vi "ExposeSetObjectMapNamepathDataToVartiant.vi"(0 "Value In (or type, reference)":refnum<data-value>, 1 "MatlabDataBundle":T1, 2 "NamePath":string[](array[string]), 3 "Namepath Index":i32, 4 "Updatied controls(s)":refnum<vi>[](array[refnum]), 6 "Allow Variant Values (f)":bool, 18 "Info":string[](array[string])) -> (14 "Value Out Ref":refnum<data-value>, 16 "Updated control(s) out":refnum<vi>[](array[refnum]))   [LabVIEW 2017]
uses:
  ExposeObjectMapNamepathData.ctl
  ExposeMapperDataTypeEnum.ctl
  ExposeObjectMapContainerTypeEnum.ctl
panel:
  out "Updating index":i32
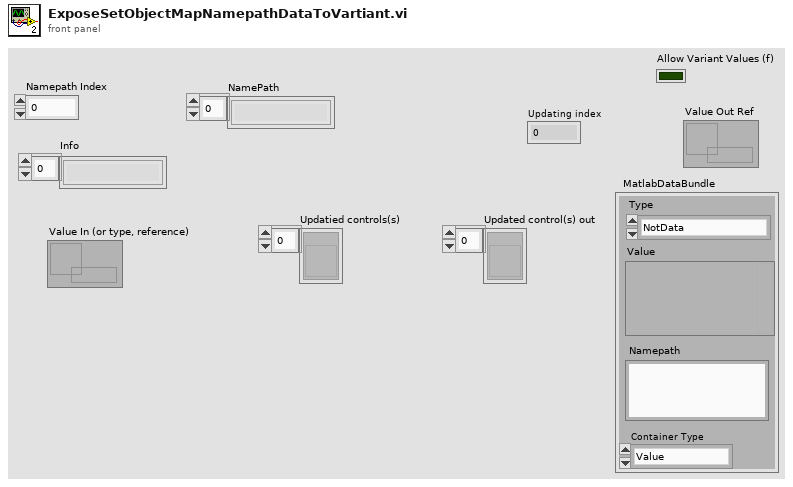
[diagram p1: front panel]
types:
  T1 = typedef "ExposeObjectMapNamepathData.ctl" = cluster{"Type":T2, "Value":variant, "Namepath":string, "Container Type":T3}
  T2 = typedef "ExposeMapperDataTypeEnum.ctl" = enum16{"NotData", "int8", "byte", "int16", "uint16", "int32", "uint32", "int64", "uint64", "Single", "Double", "String", "Boolean", "Container"}
  T3 = typedef "ExposeObjectMapContainerTypeEnum.ctl" = enum16{"Value", "Array", "Waveform", "NetContainer"}
  T4 = typedef "ExposeMapperObjectTypeEnum.ctl" = enum16{"NotAValidObject", "Value", "Variant", "Cluster", "Array", "Asng. Refnum"}
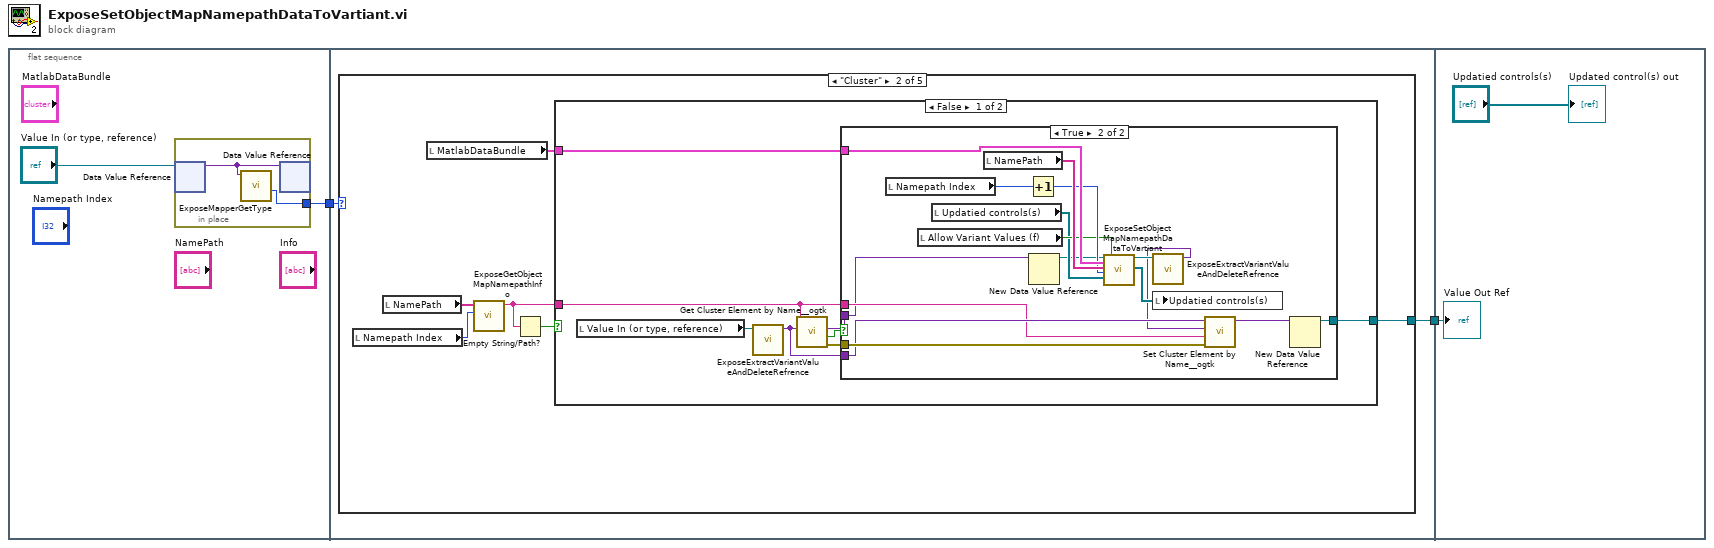
[diagram p0: block diagram]
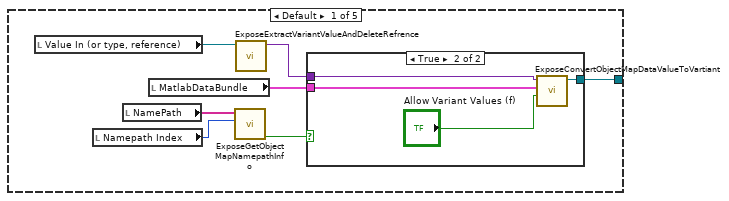
[diagram p2: hidden frame]
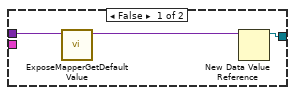
[diagram p3: hidden frame]
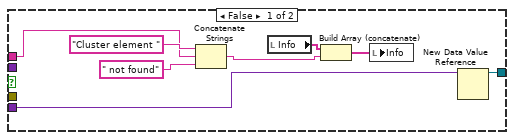
[diagram p4: hidden frame]
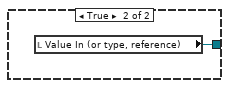
[diagram p5: hidden frame]
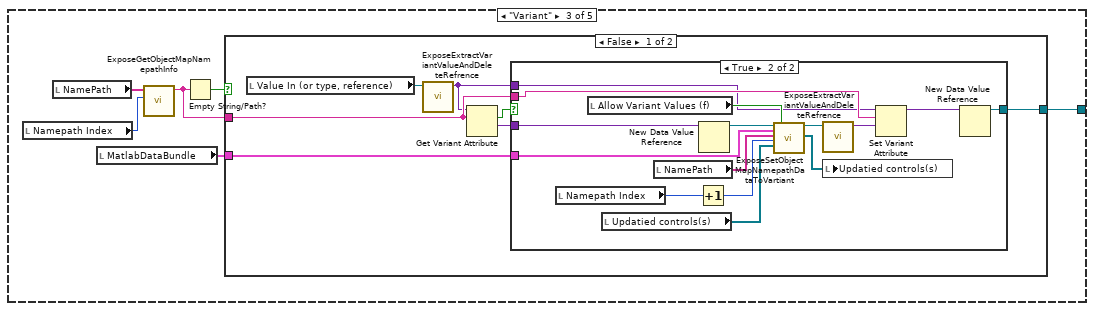
[diagram p6: hidden frame]
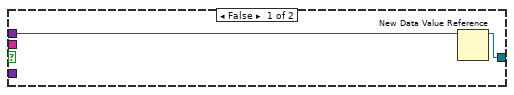
[diagram p7: hidden frame]
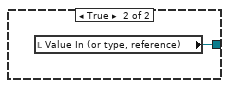
[diagram p8: hidden frame]
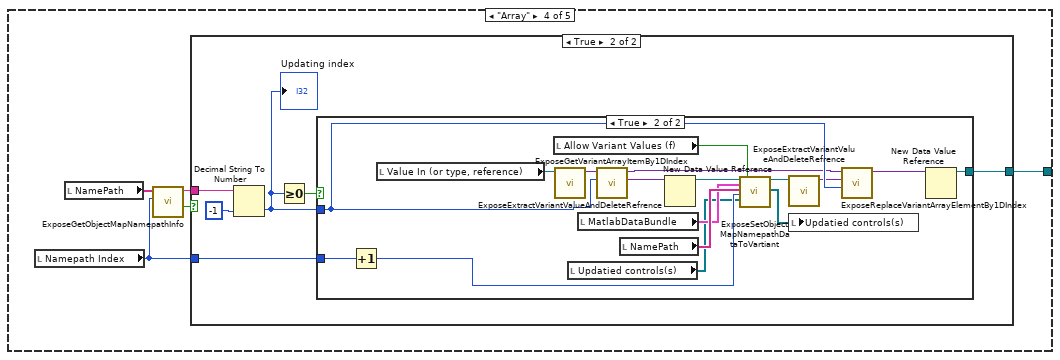
[diagram p9: hidden frame]
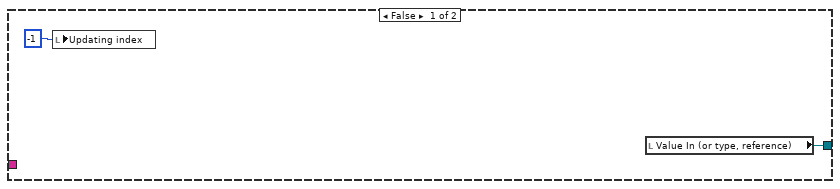
[diagram p10: hidden frame]
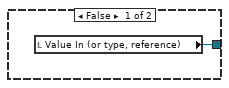
[diagram p11: hidden frame]
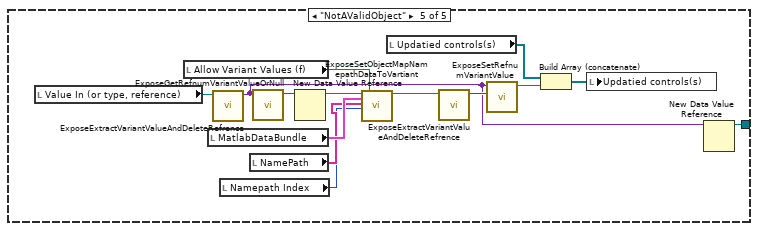
[diagram p12: hidden frame]
diagram:
  n1 = flat-sequence {
    tunnel: [w3] -> w2
    tunnel: w2 -> [w8]
    tunnel: [w7] -> w1
    tunnel: w1 -> [w138]
    frame #0 {
      n2 = in-place {
        in-place-border: [w6] -> w3
        n3 = in-place-dvr #1("Value In (or type, reference)") -> (w5:variant)  [unwired: 1 out]
        n4 = call "ExposeMapperGetType.vi"("Value"=w5) -> ("OType"=w6:T4)  [unwired: 5 in, 5 out]
        n5 = in-place-dvr #1(w5) -> ()  [unwired: 2 out]
      }
    }
    frame #1 {
      n6 = case shown="\"Cluster\"" w8 {
        tunnel: [w11 w23 w62 w93 w126] -> w7
        frame Default {
          n7 = local read "Value In (or type, reference)"() -> (w10:refnum<data-value>)
          n8 = local read "Namepath Index"() -> (w14:i32)
          n9 = local read "NamePath"() -> (w13:string[])
          n10 = local read "MatlabDataBundle"() -> (w15:T1)
          n11 = call "ExposeGetObjectMapNamepathInfo.vi"("Namepath Index"=w14, "NamePath"=w13) -> ("At path end"=w12:bool)  [unwired: 7 in, 2 out]
          n12 = call "ExposeExtractVariantValueAndDeleteRefrence.vi"("Data Value Reference in"=w10) -> ("Value out"=w9:variant)  [unwired: 10 in]
          n13 = case shown="True" w12 {
            tunnel: w9 -> [w18 w22]
            tunnel: w15 -> [_ w21]
            tunnel: [w16 w19] -> w11
            frame False {
              n14 = call "ExposeMapperGetDefaultValue.vi"("From Value Type"=w18) -> ("Default Value"=w17:variant)  [unwired: 10 in]
              n15 = New Data Value Reference(data value=w17) -> (data value reference=w16:refnum<data-value>)  [unwired: 1 in, 1 out]
            }
            frame True {
              n16 = call "ExposeConvertObjectMapDataValueToVartiant.vi"("Allow Variant Values (f)"="Allow Variant Values (f)", "NamepathData"=w21, "Data Value"=w22) -> ("Value Ref"=w19:refnum<data-value>)  [unwired: 8 in]
            }
          }
        }
        frame "Cluster" {
          n17 = local read "Namepath Index"() -> (w24:i32)
          n18 = local read "NamePath"() -> (w26:string[])
          n19 = local read "MatlabDataBundle"() -> (w28:T1)
          n20 = call "ExposeGetObjectMapNamepathInfo.vi"("Namepath Index"=w24, "NamePath"=w26) -> ("Name"=w25:string)  [unwired: 7 in, 2 out]
          n21 = Empty String/Path?(string/path=w25) -> (empty?=w27:bool)
          n22 = case shown="False" w27 {
            tunnel: w28 -> [w35 _]
            tunnel: w25 -> [w33 _]
            tunnel: [w31 w61] -> w23
            frame False {
              n23 = local read "Value In (or type, reference)"() -> (w30:refnum<data-value>)
              n24 = call "ExposeExtractVariantValueAndDeleteRefrence.vi"("Data Value Reference in"=w30) -> ("Value out"=w29:variant)  [unwired: 10 in]
              n25 = call <userlib>:"Get Cluster Element by Name__ogtk.vi"("Element Name"=w33, "Cluster"=w29) -> ("error out"=w34:errorcluster, "found?"=w32:bool, "VElement"=w36:variant)  [unwired: 7 in]
              n26 = case shown="True" w32 {
                tunnel: w36 -> [_ w46]
                tunnel: w35 -> [_ w60]
                tunnel: w34 -> [_ w59]
                tunnel: w29 -> [w37 w58]
                tunnel: w33 -> [w41 w57]
                tunnel: [w38 w47] -> w31
                frame False {
                  n27 = Concatenate Strings("Cluster element ", w41, " not found") -> (w43:string)
                  n28 = local read "Info"() -> (w44:string[])
                  n29 = Build Array (concatenate)(w44, w43) -> (w39:string[])
                  n30 = local write "Info"(w39) -> ()
                  n31 = New Data Value Reference(data value=w37) -> (data value reference=w38:refnum<data-value>)  [unwired: 1 in, 1 out]
                }
                frame True {
                  n32 = local read "Namepath Index"() -> (w55:i32)
                  n33 = local read "Allow Variant Values (f)"() -> (w53:bool)
                  n34 = local read "Updatied controls(s)"() -> (w52:refnum<vi>[])
                  n35 = local read "NamePath"() -> (w56:string[])
                  n36 = Increment(x=w55) -> (x+1=w54:i32)
                  n37 = New Data Value Reference(data value=w46) -> (data value reference=w45:refnum<data-value>)  [unwired: 1 in, 1 out]
                  n38 = call "ExposeSetObjectMapNamepathDataToVartiant.vi"("Value In (or type, reference)"=w45, "MatlabDataBundle"=w60, "NamePath"=w56, "Namepath Index"=w54, "Updatied controls(s)"=w52, "Allow Variant Values (f)"=w53) -> ("Value Out Ref"=w50:refnum<data-value>, "Updated control(s) out"=w51:refnum<vi>[])  [unwired: 12 in]
                  n39 = call "ExposeExtractVariantValueAndDeleteRefrence.vi"("Data Value Reference in"=w50) -> ("Value out"=w49:variant)  [unwired: 10 in]
                  n40 = local write "Updatied controls(s)"(w51) -> ()
                  n41 = call <userlib>:"Set Cluster Element by Name__ogtk.vi"("error in (no error)"=w59, "Element Name (\"\": New Element Data Name)"=w57, "New Element Value"=w49, "Cluster"=w58) -> ("VCluster out"=w48:variant)  [unwired: 5 in, 2 out]
                  n42 = New Data Value Reference(data value=w48) -> (data value reference=w47:refnum<data-value>)  [unwired: 1 in, 1 out]
                }
              }
            }
            frame True {
              n43 = local read "Value In (or type, reference)"() -> (w61:refnum<data-value>)
            }
          }
        }
        frame "Variant" {
          n44 = local read "Namepath Index"() -> (w63:i32)
          n45 = local read "NamePath"() -> (w65:string[])
          n46 = local read "MatlabDataBundle"() -> (w67:T1)
          n47 = call "ExposeGetObjectMapNamepathInfo.vi"("Namepath Index"=w63, "NamePath"=w65) -> ("Name"=w64:string)  [unwired: 7 in, 2 out]
          n48 = Empty String/Path?(string/path=w64) -> (empty?=w66:bool)
          n49 = case shown="False" w66 {
            tunnel: w67 -> [w74 _]
            tunnel: w64 -> [w73 _]
            tunnel: [w70 w92] -> w62
            frame False {
              n50 = local read "Value In (or type, reference)"() -> (w69:refnum<data-value>)
              n51 = call "ExposeExtractVariantValueAndDeleteRefrence.vi"("Data Value Reference in"=w69) -> ("Value out"=w68:variant)  [unwired: 10 in]
              n52 = Get Variant Attribute(Variant=w68, name=w73) -> (found=w71:bool, value=w72:variant)  [unwired: 2 in, 2 out]
              n53 = case shown="True" w71 {
                tunnel: w72 -> [_ w78]
                tunnel: w74 -> [_ w91]
                tunnel: w73 -> [_ w86]
                tunnel: [w76 w79] -> w70
                tunnel: w68 -> [w75 w83]
                frame False {
                  n54 = New Data Value Reference(data value=w75) -> (data value reference=w76:refnum<data-value>)  [unwired: 1 in, 1 out]
                }
                frame True {
                  n55 = local read "Namepath Index"() -> (w89:i32)
                  n56 = local read "Allow Variant Values (f)"() -> (w87:bool)
                  n57 = local read "Updatied controls(s)"() -> (w85:refnum<vi>[])
                  n58 = local read "NamePath"() -> (w90:string[])
                  n59 = Increment(x=w89) -> (x+1=w88:i32)
                  n60 = New Data Value Reference(data value=w78) -> (data value reference=w77:refnum<data-value>)  [unwired: 1 in, 1 out]
                  n61 = call "ExposeSetObjectMapNamepathDataToVartiant.vi"("Value In (or type, reference)"=w77, "MatlabDataBundle"=w91, "NamePath"=w90, "Namepath Index"=w88, "Updatied controls(s)"=w85, "Allow Variant Values (f)"=w87) -> ("Value Out Ref"=w82:refnum<data-value>, "Updated control(s) out"=w84:refnum<vi>[])  [unwired: 12 in]
                  n62 = call "ExposeExtractVariantValueAndDeleteRefrence.vi"("Data Value Reference in"=w82) -> ("Value out"=w81:variant)  [unwired: 10 in]
                  n63 = local write "Updatied controls(s)"(w84) -> ()
                  n64 = Set Variant Attribute(Variant=w83, name=w86, value=w81) -> (Variant out=w80:variant)  [unwired: 1 in, 2 out]
                  n65 = New Data Value Reference(data value=w80) -> (data value reference=w79:refnum<data-value>)  [unwired: 1 in, 1 out]
                }
              }
            }
            frame True {
              n66 = local read "Value In (or type, reference)"() -> (w92:refnum<data-value>)
            }
          }
        }
        frame "Array" {
          n67 = local read "Namepath Index"() -> (w97:i32)
          n68 = local read "NamePath"() -> (w96:string[])
          n69 = call "ExposeGetObjectMapNamepathInfo.vi"("Namepath Index"=w97, "NamePath"=w96) -> ("Namepart found?"=w94:bool, "Name"=w95:string)  [unwired: 7 in, 1 out]
          n70 = case shown="True" w94 {
            tunnel: w97 -> [_ w102]
            tunnel: w95 -> [_ w101]
            tunnel: [w98 w100] -> w93
            frame False {
              n71 = local write "Updating index"(-1 ("Updating index")) -> ()
              n72 = local read "Value In (or type, reference)"() -> (w98:refnum<data-value>)
            }
            frame True {
              n73 = Decimal String To Number(string=w101, default (0L)=-1 ("default (0 I32)")) -> (number=w104:i32)  [unwired: 1 in, 1 out]
              "Updating index" <- w104
              n74 = Greater Or Equal To 0?(x=w104) -> (x >= 0?=w103:bool)
              n75 = case shown="True" w103 {
                tunnel: w104 -> [_ w119]
                tunnel: w102 -> [_ w121]
                tunnel: [w106 w110] -> w100
                frame False {
                  n76 = local read "Value In (or type, reference)"() -> (w106:refnum<data-value>)
                }
                frame True {
                  n77 = Increment(x=w121) -> (x+1=w120:i32)
                  n78 = local read "Value In (or type, reference)"() -> (w115:refnum<data-value>)
                  n79 = local read "Allow Variant Values (f)"() -> (w118:bool)
                  n80 = call "ExposeExtractVariantValueAndDeleteRefrence.vi"("Data Value Reference in"=w115) -> ("Value out"=w114:variant)  [unwired: 10 in]
                  n81 = local read "Updatied controls(s)"() -> (w117:refnum<vi>[])
                  n82 = local read "MatlabDataBundle"() -> (w122:T1)
                  n83 = call "ExposeGetVariantArrayItemBy1DIndex.vi"("Index"=w119, "Array in"=w114) -> ("Array Element"=w108:variant, "Array out"=w109:variant)  [unwired: 8 in]
                  n84 = local read "NamePath"() -> (w123:string[])
                  n85 = New Data Value Reference(data value=w108) -> (data value reference=w107:refnum<data-value>)  [unwired: 1 in, 1 out]
                  n86 = call "ExposeSetObjectMapNamepathDataToVartiant.vi"("Value In (or type, reference)"=w107, "MatlabDataBundle"=w122, "NamePath"=w123, "Namepath Index"=w120, "Updatied controls(s)"=w117, "Allow Variant Values (f)"=w118) -> ("Value Out Ref"=w113:refnum<data-value>, "Updated control(s) out"=w116:refnum<vi>[])  [unwired: 12 in]
                  n87 = call "ExposeExtractVariantValueAndDeleteRefrence.vi"("Data Value Reference in"=w113) -> ("Value out"=w112:variant)  [unwired: 10 in]
                  n88 = local write "Updatied controls(s)"(w116) -> ()
                  n89 = call "ExposeReplaceVariantArrayElementBy1DIndex.vi"("Index (1D)"=w119, "Value"=w112, "Array in"=w109) -> ("Array out"=w111:variant)  [unwired: 8 in]
                  n90 = New Data Value Reference(data value=w111) -> (data value reference=w110:refnum<data-value>)  [unwired: 1 in, 1 out]
                }
              }
            }
          }
        }
        frame "NotAValidObject" {
          n91 = local read "Value In (or type, reference)"() -> (w130:refnum<data-value>)
          n92 = local read "Allow Variant Values (f)"() -> (w134:bool)
          n93 = local read "MatlabDataBundle"() -> (w137:T1)
          n94 = call "ExposeExtractVariantValueAndDeleteRefrence.vi"("Data Value Reference in"=w130) -> ("Value out"=w127:variant)  [unwired: 10 in]
          n95 = local read "Namepath Index"() -> (w135:i32)
          n96 = local read "NamePath"() -> (w136:string[])
          n97 = call "ExposeGetRefnumVariantValueOrNull.vi"("ControlVariant"=w127) -> ("Value"=w125:variant)  [unwired: 8 in, 2 out]
          n98 = New Data Value Reference(data value=w125) -> (data value reference=w124:refnum<data-value>)  [unwired: 1 in, 1 out]
          n99 = call "ExposeSetObjectMapNamepathDataToVartiant.vi"("Value In (or type, reference)"=w124, "MatlabDataBundle"=w137, "NamePath"=w136, "Namepath Index"=w135, "Allow Variant Values (f)"=w134) -> ("Value Out Ref"=w129:refnum<data-value>)  [unwired: 13 in, 1 out]
          n100 = local read "Updatied controls(s)"() -> (w131:refnum<vi>[])
          n101 = call "ExposeExtractVariantValueAndDeleteRefrence.vi"("Data Value Reference in"=w129) -> ("Value out"=w128:variant)  [unwired: 10 in]
          n102 = call "ExposeSetRefnumVariantValue.vi"("Value"=w128, "ControlVariant"=w127) -> ("Control"=w133:refnum<vi>)  [unwired: 8 in, 1 out]
          n103 = Build Array (concatenate)(w131, w133) -> (w132:refnum<vi>[])
          n104 = local write "Updatied controls(s)"(w132) -> ()
          n105 = New Data Value Reference(data value=w127) -> (data value reference=w126:refnum<data-value>)  [unwired: 1 in, 1 out]
        }
      }
    }
    frame #2 {
      "Updated control(s) out" <- "Updatied controls(s)"
      "Value Out Ref" <- w138
    }
  }
